vi "_OLS_5PtCalibration.vi"() -> ()   [LabVIEW 2024]
uses:
  Control Definitions/Def_PumpSpeed.ctl
  Control Definitions/DEF_CalConstants.ctl
  Control Definitions/Def PumpCtlRefs.ctl
  Control Definitions/Def CalTable.ctl
  Control Definitions/Def CalCoef.ctl
  Control Definitions/Def_LevelCalCoef.ctl
  Control Definitions/Registry Keys.ctl
  Control Definitions/Global 2.vi
  Control Definitions/Global 1.vi
  Control Definitions/DEF_5ptCalState.ctl
panel:
  out "Laser (raw) 2":dbl=-0.0 format="%#_4g"
  out "Numeric":i32
  out "Cal Coef":T1={"Level"={"M"=-0.9990777034816695, "B"=9.617362923679963, "Mc"=-1.0009231479344565, "Bc"=9.626241172397878, "LMe"=7.844}, "Dataq Ch"=[{"B"=-0.34241100677002123, "M"=175.4094780519764}, {"B"=-0.7865736704446391, "M"=174.89102005231038}]}
  in  "Default Cal Table":T3={"Level"={"LSf"=2.6, "LMf"=3.511, "LKf"=6.112, "LMe"=7.844, "LKe"=1.775, "LSe"=8.0}, "DataQ CH"=[{"RqLA"=0.592, "RmLA"=103.5, "RqHA"=5.171, "RmHA"=906.7}, {"RqLA"=0.582, "RmLA"=101.0, "RqHA"=5.17, "RmHA"=903.4}]}
  out "ItemPath":string
  in  "End Prog":bool
  out "PumpCtlRef out":T4
  out "Reg Cal Constants":T5={"Measure High"="3.125", "Laser High"="6.534", "Measure Low"="7.483", "Laser Low"="2.877", "Cal Name"="Rick A", "Cal Date"="8/22/2024 8:52:33 AM", "Empty Inches"=8.0, "Full Inches"=2.6, "Valid"=FALSE}
  in  "Pump Speed":T6=enum."STOP"
  in  "Num Chan":i32=2
  in  "VISA Refnum in":refnum<visa-resource-name>="COM3"
  in  "SimPV":bool
  out "Root Path":path=path "C:/AllenProjects/PWC-OLS"
  out "Time(ms)":dbl=1094.5499999995523
  out "Level":bool
  out "DataQ":bool
  in  "ChA":dbl(slide)=24.489795918367346 scale=0.0..1200.0
  in  "ChB":dbl(slide)=36.73469387755102 scale=0.0..1200.0
  in  "ChB +100":bool
  in  "ChA +100":bool
  in  "Check":bool
  out "Laser (raw)":dbl=-0.0 format="%#_4g"
  in  "DUT":i16=1
  in  "Pump JOG":bool=TRUE
  in  "Run Test":bool
  in  "Normal":cluster{u32, u32}[](array[cluster])=[{16711680, 1244948}]
  out "Level \nStatus":bool
  out "DataQ\nStatus":bool
  in  "Level SP":dbl(slide)=8.0 scale=8.5..2.0
  in  "Level PV":dbl(slide)=9.617362923679963 scale=8.5..2.0
  out "Level":dbl=9.617362923679963 format="%.3f"
  in  "Drain":bool
  in  "Fill":bool
  in  "Simulate":bool
  out "TEST NME":string="OLR001--"
  out "DataQ Input":T7(graph)={"ChA Ohms"=24.489795918367346, "ChB Ohms"=36.73469387755102, "Laser (raw)"=-0.0}
  out "Time Stamp":timestamp=timestamp(3809961154.032212 s since 1904-01-01)
  in  "stop":bool
  out "ChB Ohms":dbl=36.73469387755102 format="%.1f"
  out "ChA Ohms":dbl=24.489795918367346 format="%.1f"
  # "Calibration & Scaling Table\n               Tank         Key          Ref\n               Scale        Level        Measure\nEmpty\n\n\nFull"
  # "8.0      1.7752      7.844\n\n2.6      6.112        3.511"
  # "CHA"
  # "CHB"
  # "ATP       Resistance     Fill        Drain"
  # "ATP       Resistance     Fill        Drain"
  # "Simulated Instrument Inputs"
  # "PUMP"
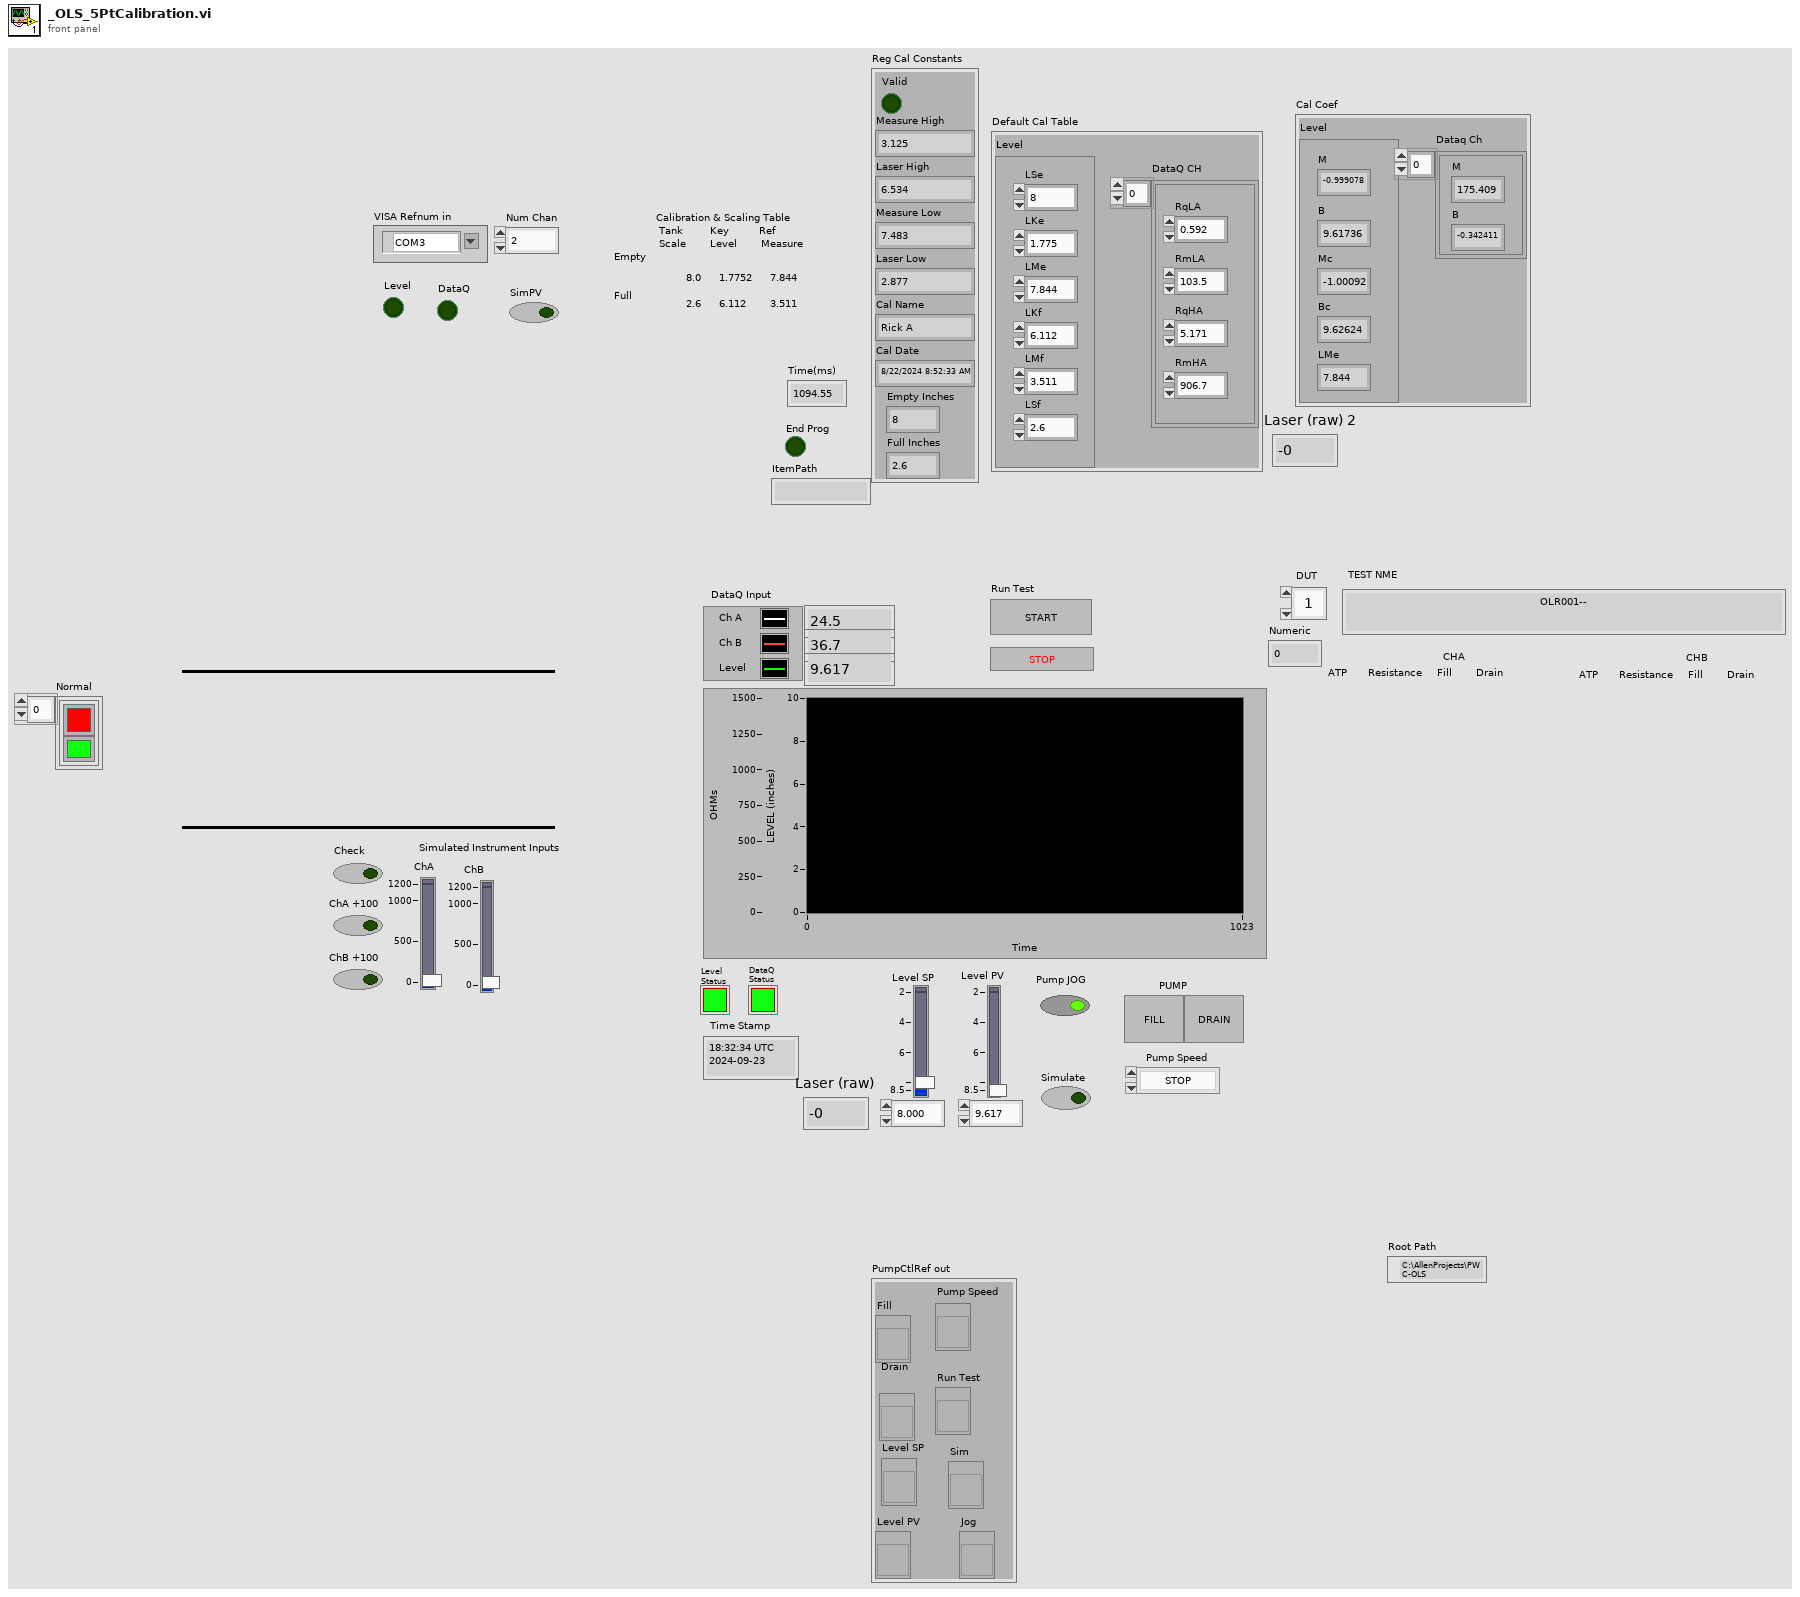
[diagram p1: front panel]
types:
  T1 = typedef "Def CalCoef.ctl" = cluster{"Level":T2, "Dataq Ch":cluster{"B":dbl, "M":dbl}[]}
  T2 = typedef "Def_LevelCalCoef.ctl" = cluster{"M":dbl, "B":dbl, "Mc":dbl, "Bc":dbl, "LMe":dbl}
  T3 = typedef "Def CalTable.ctl" = cluster{"Level":cluster{"LSf":dbl, "LMf":dbl, "LKf":dbl, "LMe":dbl, "LKe":dbl, "LSe":dbl}, "DataQ CH":cluster{"RqLA":dbl, "RmLA":dbl, "RqHA":dbl, "RmHA":dbl}[]}
  T4 = typedef "Def PumpCtlRefs.ctl" = cluster{"Fill ":refnum<vi>, "Drain":refnum<vi>, "Level PV":refnum<vi>, "Pump Speed":refnum<vi>, "Run Test":refnum<vi>, "Sim":refnum<vi>, "Jog":refnum<vi>, "Level SP":refnum<vi>}
  T5 = typedef "DEF_CalConstants.ctl" = cluster{"Measure High":string, "Laser High":string, "Measure Low":string, "Laser Low":string, "Cal Name":string, "Cal Date":string, "Empty Inches":dbl, "Full Inches":dbl, "Valid":bool}
  T6 = typedef "Def_PumpSpeed.ctl" = enum16{"FAST", "SLOW", "CREEP", "STOP"}
  T7 = cluster{"ChA Ohms":dbl, "ChB Ohms":dbl, "Laser (raw)":dbl}
  T8 = typedef "Registry Keys.ctl" = enum16{"Report Files Key", "Config Files Key"}
  T9 = cluster{"Level \nStatus":refnum<vi>, "DataQ\nStatus":refnum<vi>}
  T10 = typedef "Def FullCfg.ctl" = cluster{"Bench Config":T11, "Test Value Table ":dbl[][], "Table Col Titles":string[][], "cluster":T4, "Bench Status":T12}
  T11 = typedef "Def BenchCfg.ctl" = cluster{"Name":string, cluster{"Step Levels":dbl, "Tolerance":dbl, "Sample Rate":dbl, "Resistor":dbl, "M Level Cal":dbl, "[B Level Cal":dbl, "Max Fill Rate":dbl, "Empty Inches":dbl, "Full Inches":dbl}}
  T12 = typedef "Def Bench Status.ctl" = cluster{"Pump Status":refnum<vi>, "Instrumnet\n Status":refnum<vi>}
  T13 = typedef "DEF_5ptCalState.ctl" = enum16{"Start", "Load Tester", "Go Auto", "Level 1", "Reveiw ", "Save", "Exit"}
  T14 = cluster{"Resistor":dbl, "Fill":dbl, "Drain":dbl, "Status":i16}
  T15 = cluster{"Resistor":dbl, "Fill":dbl, "Drain":dbl, "Status":i16}[][]
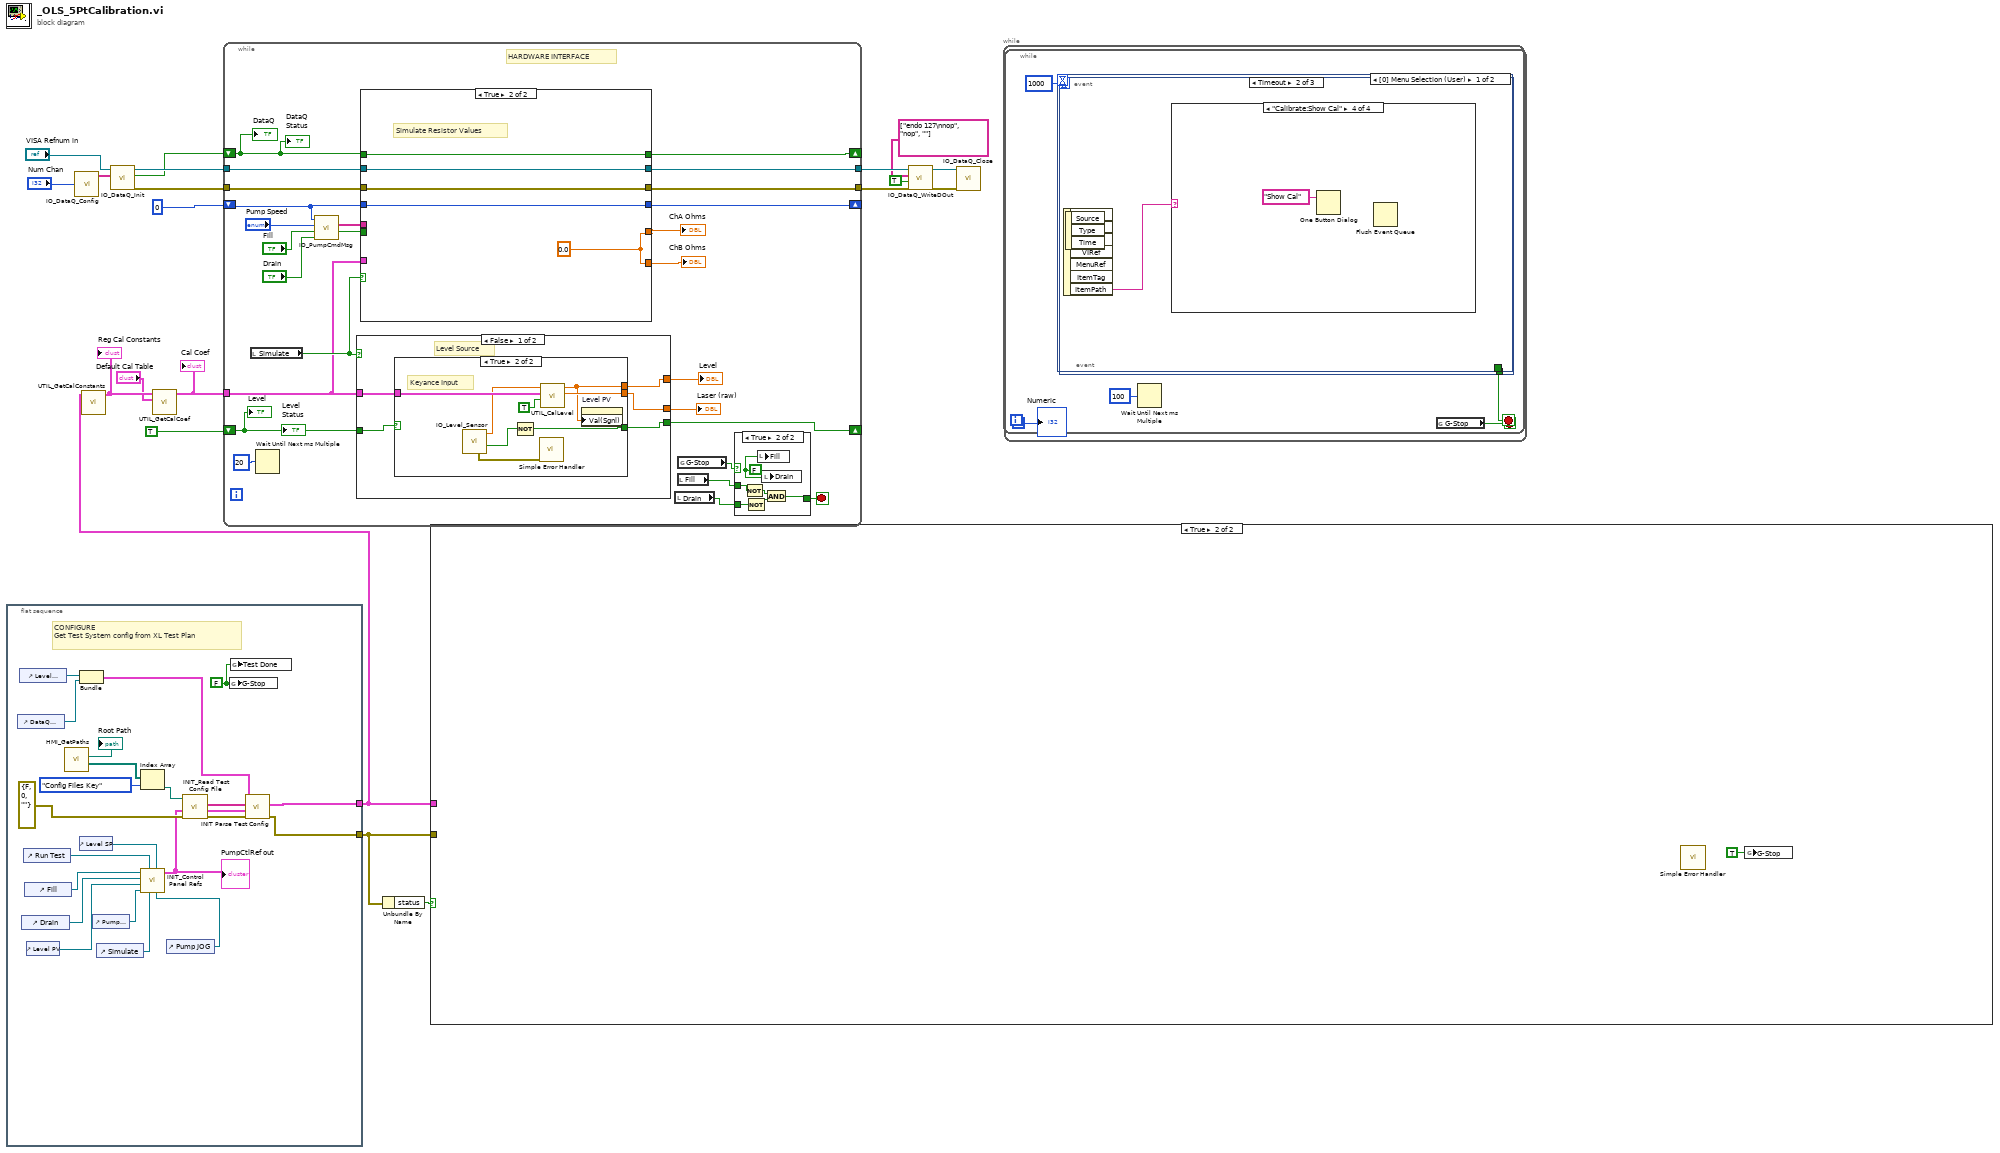
[diagram p0: block diagram]
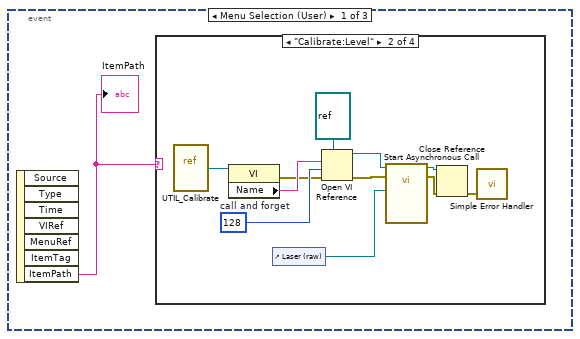
[diagram p2: hidden frame]
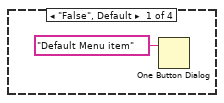
[diagram p3: hidden frame]
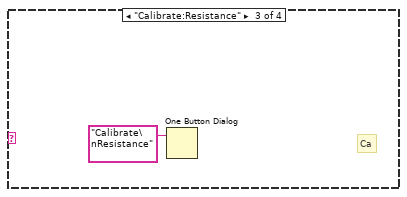
[diagram p4: hidden frame]
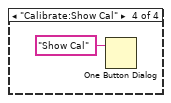
[diagram p5: hidden frame]
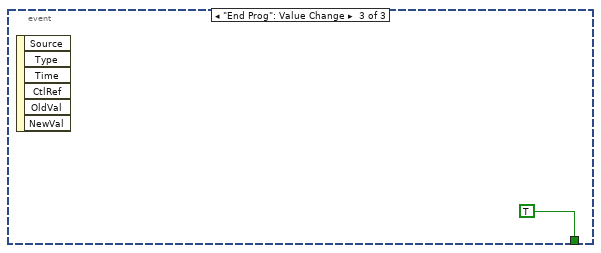
[diagram p6: hidden frame]
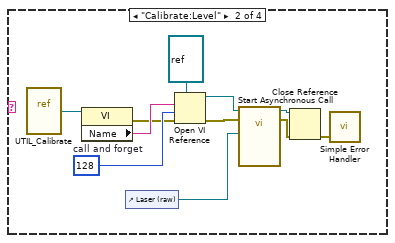
[diagram p8: hidden frame]
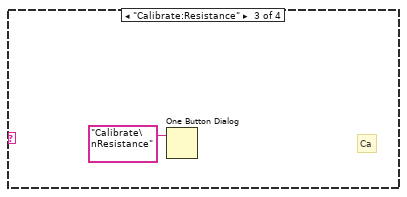
[diagram p9: hidden frame]
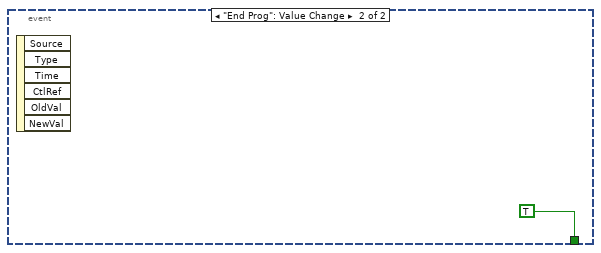
[diagram p10: hidden frame]
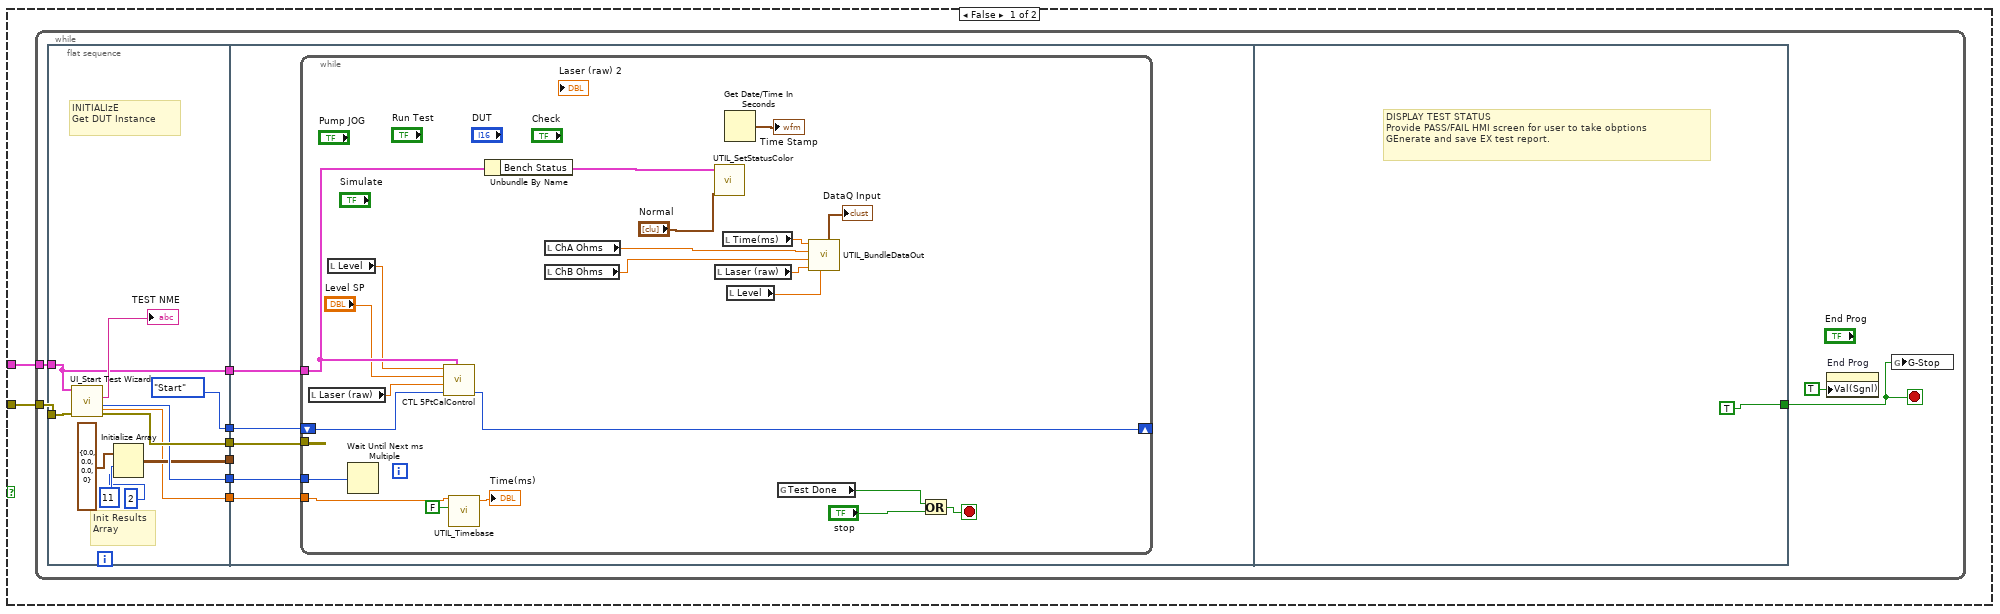
[diagram p11: hidden frame]
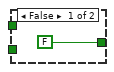
[diagram p12: hidden frame]
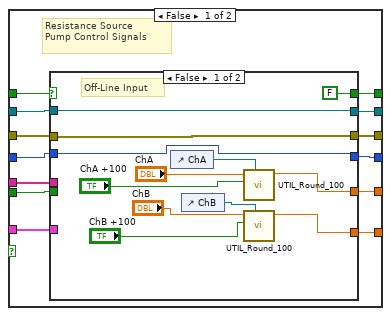
[diagram p13: hidden frame]
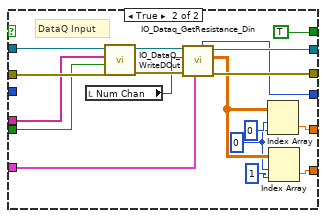
[diagram p14: hidden frame]
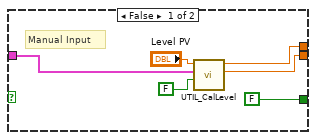
[diagram p15: hidden frame]
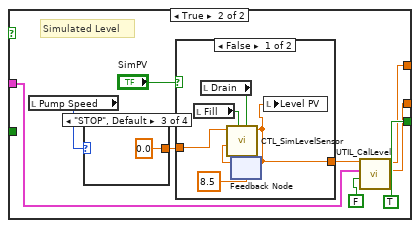
[diagram p16: hidden frame]
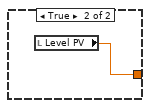
[diagram p17: hidden frame]
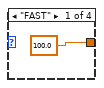
[diagram p18: hidden frame]
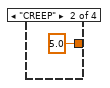
[diagram p19: hidden frame]
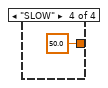
[diagram p20: hidden frame]
diagram:
  n1 = flat-sequence {
    tunnel: [w40] -> w14
    tunnel: [w32] -> w3
    frame #0 {
      w27 = FALSE ("G-Stop")
      # "CONFIGURE\nGet Test System config from XL Test Plan"
      n2 = control-ref of="DataQ\nStatus"() -> (w29:refnum<vi>)
      n3 = control-ref of="Level \nStatus"() -> (w39:refnum<vi>)
      n4 = control-ref of="Drain"() -> (w41:refnum<vi>)
      n5 = control-ref of="Run Test"() -> (w34:refnum<vi>)
      n6 = control-ref of="Fill"() -> (w35:refnum<vi>)
      n7 = control-ref of="Level PV"() -> (w37:refnum<vi>)
      n8 = call "HMI_GetPaths.vi"() -> ("Default Paths"=w22:path[], "Root Path"=→"Root Path":path)  [unwired: 10 in]
      n9 = Bundle("Level \nStatus"=w39, "DataQ\nStatus"=w29) -> (w38:T9)  [unwired: 1 in]
      n10 = control-ref of="Level SP"() -> (w28:refnum<vi>)
      n11 = control-ref of="Pump Speed"() -> (w24:refnum<vi>)
      n12 = control-ref of="Simulate"() -> (w31:refnum<vi>)
      n13 = Index Array(array=w22, index=Registry_Keys."Config Files Key" ("Reg Key")) -> (element=w21:path)
      n14 = control-ref of="Pump JOG"() -> (w30:refnum<vi>)
      n15 = call "INIT_Control Panel Refs.vi"("Jog"=w30, "Level SP"=w28, "Sim"=w31, "Run Test"=w34, "Pump Speed"=w24, "Level PV"=w37, "Drain"=w41, "Fill"=w35) -> ("PumpCtlRef out"=w25:T4)  [unwired: 3 in]
      "PumpCtlRef out" <- w25
      n16 = call "INIT_Read Test Config File.vi"("error in (no error)"=errorcluster {"status"=FALSE, "code"=0, "source"=""}, "Path"=w21) -> ("error out 2"=w33:errorcluster, "Config\nFile Data"=w36:string[][])  [unwired: 8 in]
      n17 = global write "Global 1.vi" "G-Stop"(w27) -> ()
      n18 = global write "Global 2.vi" "Test Done"(w27) -> ()
      n19 = call "INIT Parse Test Config.vi"("error in (no error)"=w33, "Pump CtlRef In"=w25, "All XL Input"=w36, "Bench Status"=w38) -> ("error out"=w40:errorcluster, "Full Config"=w32:T10)  [unwired: 5 in, 1 out]
    }
  }
  n20 = call "IO_DataQ_Config.vi"("Num Chan"="Num Chan") -> ("Init Message"=w20:string[])  [unwired: 10 in]
  n21 = call "UTIL_GetCalConstants.vi"("Full Config"=w3) -> ("Cal Constants"=w4:T5)  [unwired: 9 in, 1 out]
  "Reg Cal Constants" <- w4
  n22 = call "IO_DataQ_Init.vi"("Command\nList"=w20, "VISA Refnum in"="VISA Refnum in") -> ("error out"=w18:errorcluster, "Connected?"=w17:bool, "VISA resource name out"=w19:refnum<visa-resource-name>)  [unwired: 7 in]
  n23 = call "UTIL_GetCalCoef.vi"("Cal Table"="Default Cal Table", "Cal Constants"=w4) -> ("Cal Coef"=w1:T1)  [unwired: 9 in]
  "Cal Coef" <- w1
  n24 = while {
    shift-right: [w65] -> _
    shift-left: TRUE ("Pump \nStatus") -> [w47]
    tunnel: w19 -> [w64]
    tunnel: w18 -> [w63]
    tunnel: [w61] -> w13
    tunnel: [w62] -> w11
    shift-right: [w60] -> _
    shift-left: w17 -> [w59]
    tunnel: w1 -> [w43]
    shift-right: [w50] -> _
    shift-left: 0 -> [w46]
    stop <- w55 stop-if-true
    # "HARDWARE INTERFACE"
    n25 = local read "Simulate"() -> (w57:bool)
    n26 = Wait Until Next ms Multiple(millisecond multiple=u32 20) -> ()  [unwired: 1 out]
    n27 = call "IO_PumpCmdMsg.vi"("Drain Signal"="Drain", "FIll Signal"="Fill", "Pump Speed"="Pump Speed", "Cmd IN"=w46) -> ("Msg Active"=w44:bool, "Message"=w58:string[])  [unwired: 4 in, 2 out]
    n28 = case shown="False" w57 {
      tunnel: [w128 w148] -> w45
      tunnel: [w127 w150] -> w66
      tunnel: [w124 TRUE] -> w65
      tunnel: w47 -> [w126 _]
      tunnel: w43 -> [w125 w143]
      frame False {
        # "Level Source"
        n29 = case shown="True" w126 {
          tunnel: [w132 w135] -> w128
          tunnel: [w131 w140] -> w127
          tunnel: [FALSE ("status") w139] -> w124
          tunnel: w125 -> [w133 w141]
          frame False {
            # "Manual Input"
            n30 = call "UTIL_CalLevel.vi"("Key is In?"=FALSE, "Cal Coef"=w133, "Input"="Level PV") -> ("PVc"=w131:dbl, "PVs"=w132:dbl)  [unwired: 7 in]
          }
          frame True {
            # "Keyance Input"
            n31 = call "IO_Level_Sensor.vi"() -> ("status"=w137:bool, "PV (raw)"=w138:dbl, "error OUT"=w136:errorcluster)  [unwired: 9 in]
            n32 = Not(x=w137) -> (.not. x?=w139:bool)
            n33 = call <vilib>:"Simple Error Handler.vi"("error in (no error)"=w136) -> ()  [unwired: 4 in, 5 out]
            n34 = call "UTIL_CalLevel.vi"("Key is In?"=TRUE, "Cal Coef"=w141, "Input"=w138) -> ("PVc"=w140:dbl, "PVs"=w135:dbl)  [unwired: 7 in]
            n35 = property on="Level PV" class="Slide (strict)"("Val(Sgnl)"=w135) -> ()  [unwired: 2 in, 2 out]
          }
        }
      }
      frame True {
        # "Simulated Level"
        n36 = local read "Pump Speed"() -> (w146:T6)
        n37 = case shown="\"STOP\", Default" w146 {
          tunnel: [100.0 ("Ctl Sig") 5.0 ("Ctl Sig") 0.0 ("Ctl Sig") 50.0 ("Ctl Sig")] -> w147
          frame "FAST" {
          }
          frame "CREEP" {
          }
          frame "STOP", Default {
          }
          frame "SLOW" {
          }
        }
        n38 = case shown="False" "SimPV" {
          tunnel: w147 -> [w156 _]
          tunnel: [w152 w158] -> w145
          frame False {
            n39 = local read "Fill"() -> (w157:bool)
            n40 = local read "Drain"() -> (w153:bool)
            n41 = feedback #1(8.5 ("PV Level Inch")) -> (w154:dbl)
            n42 = call "CTL_SimLevelSensor.vi"("Drain IN"=w153, "Fill IN"=w157, "Level PV in"=w154, "Pump Speed"=w156) -> ("PV Level Inch"=w152:dbl)  [unwired: 7 in]
            n43 = feedback-in #1(w152) -> ()
            n44 = local write "Level PV"(w152) -> ()
          }
          frame True {
            n45 = local read "Level PV"() -> (w158:dbl)
          }
        }
        n46 = call "UTIL_CalLevel.vi"("Key is In?"=FALSE, "Cal Coef"=w143, "Input"=w145) -> ("PVc"=w150:dbl, "PVs"=w148:dbl)  [unwired: 7 in]
      }
    }
    "Level" <- w45
    "Laser (raw)" <- w66
    n47 = case shown="True" w57 {
      tunnel: [w88 w119] -> w67
      tunnel: [w87 w119] -> w48
      tunnel: w64 -> [w80 w122]
      tunnel: w63 -> [w82 w121]
      tunnel: [w86 w121] -> w62
      tunnel: [w85 w122] -> w61
      tunnel: [w84 w123] -> w60
      tunnel: w59 -> [w83 w123]
      tunnel: w58 -> [w81 _]
      tunnel: w44 -> [w79 _]
      tunnel: [w78 w120] -> w50
      tunnel: w46 -> [w77 w120]
      tunnel: w43 -> [w76 _]
      frame False {
        # "Resistance Source\nPump Control Signals"
        n48 = case shown="False" w83 {
          tunnel: [w93 w115] -> w88
          tunnel: [w94 w104] -> w87
          tunnel: [w95 w118] -> w85
          tunnel: [w96 w117] -> w86
          tunnel: [FALSE TRUE] -> w84
          tunnel: w82 -> [w96 w113]
          tunnel: w81 -> [_ w109]
          tunnel: w80 -> [w95 w112]
          tunnel: w79 -> [_ w108]
          tunnel: [w89 w105] -> w78
          tunnel: w77 -> [w89 _]
          tunnel: w76 -> [_ w101]
          frame False {
            # "Off-Line Input"
            n49 = control-ref of="ChA"() -> (w92:refnum<vi>)
            n50 = control-ref of="ChB"() -> (w90:refnum<vi>)
            n51 = call "UTIL_Round_100.vi"("Num Refnum"=w92, "100"="ChA +100", "IN"="ChA") -> ("OUT"=w94:dbl)  [unwired: 8 in]
            n52 = call "UTIL_Round_100.vi"("Num Refnum"=w90, "100"="ChB +100", "IN"="ChB") -> ("OUT"=w93:dbl)  [unwired: 8 in]
          }
          frame True {
            w103 = 0 ("disabled index (col)")
            # "DataQ Input"
            n53 = local read "Num Chan"() -> (w106:i32)
            n54 = call "IO_DataQ_WriteDOut.vi"("error in (no error)"=w113, "Msg Active"=w108, "Message"=w109, "VISA Refnum in"=w112) -> ("error out"=w111:errorcluster, "VISA Refnum out"=w110:refnum<visa-resource-name>)  [unwired: 6 in]
            n55 = call "IO_Dataq_GetResistance_Din.vi"("Cal Coef"=w101, "error in (no error)"=w111, "Num Chan"=w106, "VISA Refnum in"=w110) -> ("error out"=w117:errorcluster, "Analog"=w107:dbl[][], "VISA Refnum out"=w118:refnum<visa-resource-name>, "Cmd"=w105:u32)  [unwired: 2 in, 2 out]
            n56 = Index Array(array=w107, index (row)=0 ("index"), index (col)=w103) -> (element=w104:dbl)
            n57 = Index Array(array=w107, index (row)=w103, index (col)=1 ("index")) -> (element=w115:dbl)
          }
        }
      }
      frame True {
        w119 = 0.0 ("OUT")
        # "Simulate Resistor Values"
      }
    }
    "ChA Ohms" <- w48
    "ChB Ohms" <- w67
    n58 = local read "Drain"() -> (w53:bool)
    n59 = local read "Fill"() -> (w54:bool)
    n60 = global read "Global 1.vi" "G-Stop"() -> (w56:bool)
    n61 = case shown="True" w56 {
      tunnel: [FALSE w71] -> w55
      tunnel: w54 -> [_ w73]
      tunnel: w53 -> [_ w70]
      frame False {
      }
      frame True {
        w75 = FALSE
        n62 = Not(x=w73) -> (.not. x?=w74:bool)
        n63 = Not(x=w70) -> (.not. x?=w72:bool)
        n64 = local write "Fill"(w75) -> ()
        n65 = local write "Drain"(w75) -> ()
        n66 = And(x=w74, y=w72) -> (x .and. y?=w71:bool)
      }
    }
    "DataQ\nStatus" <- w59
    "Level \nStatus" <- w47
    "DataQ" <- w59
    "Level" <- w47
  }
  n67 = Unbundle By Name(w14) -> ("status"=w16:bool)
  n68 = case shown="True" w16 {
    tunnel: w14 -> [w164 _]
    tunnel: w3 -> [w163 _]
    frame False {
      n69 = while {
        tunnel: w164 -> [w172]
        tunnel: w163 -> [w170]
        stop <- w166 stop-if-true
        n70 = flat-sequence {
          tunnel: [w183] -> w174
          tunnel: [w184] -> w173
          tunnel: w172 -> [w185]
          tunnel: [w176] -> w171
          tunnel: w170 -> [w176]
          tunnel: [DEF_5ptCalState."Start" ("Cal State In")] -> w169
          tunnel: [w178] -> w168
          tunnel: [w177] -> w167
          tunnel: w174 -> [w189]
          tunnel: w173 -> [w190]
          tunnel: w171 -> [w186]
          tunnel: w169 -> [w187]
          tunnel: w168 -> [_]
          tunnel: w167 -> [w188]
          tunnel: [TRUE] -> w166
          frame #0 {
            # "Init Results\nArray"
            # "INITIALIzE\nGet DUT Instance"
            n71 = call "UI_Start Test Wizard.vi"("error in (no error)"=w185, "Full Config"=w176) -> ("error out"=w184:errorcluster, "Time Base mS"=w183:i32, "Title"=→"TEST NME":string, "Sample Rate"=w177:dbl)  [unwired: 4 in]
            n72 = Initialize Array(T14 {"Resistor"=0.0, "Fill"=0.0, "Drain"=0.0, "Status"=0} ("Cluster 2"), 11 ("dimension size"), 2 ("dimension size")) -> (w178:T15)
          }
          frame #1 {
            n73 = while {
              tunnel: w189 -> [w211]
              tunnel: w190 -> [_]
              tunnel: w188 -> [w201]
              shift-right: [w193] -> _
              shift-left: w187 -> [w194]
              tunnel: w186 -> [w197]
              stop <- w208 stop-if-true
              n74 = local read "Laser (raw)"() -> (w191:dbl)
              n75 = local read "Level"() -> (w196:dbl)
              n76 = Wait Until Next ms Multiple(millisecond multiple=w211) -> ()  [unwired: 1 out]
              n77 = call "CTL 5PtCalControl.vi"("Full Cfg 2"=w197, "Cal State In"=w194, "Laser Raw"=w191, "Level SP"="Level SP", "Level PV"=w196) -> ("Cal State Out"=w193:T13)  [unwired: 6 in]
              n78 = call "UTIL_Timebase.vi"("Reset"=FALSE, "Sample Rate"=w201) -> ("Time(ms)"=→"Time(ms)":dbl)  [unwired: 9 in]
              n79 = Unbundle By Name(w197) -> ("Bench Status"=w209:T12)
              n80 = local read "ChA Ohms"() -> (w203:dbl)
              n81 = local read "ChB Ohms"() -> (w202:dbl)
              n82 = call "UTIL_SetStatusColor.vi"("Colors [4] in"="Normal", "Bench Status"=w209) -> ()  [unwired: 10 in]
              n83 = local read "Laser (raw)"() -> (w204:dbl)
              n84 = local read "Time(ms)"() -> (w205:dbl)
              n85 = Get Date/Time In Seconds() -> (seconds since 1Jan1904=→"Time Stamp":timestamp)
              n86 = local read "Level"() -> (w198:dbl)
              n87 = global read "Global 2.vi" "Test Done"() -> (w206:bool)
              n88 = call "UTIL_BundleDataOut.vi"("Level PV"=w198, "Laser (raw)"=w204, "ChB Ohms"=w202, "ChA Ohms"=w203, "Time (ms)"=w205) -> ("Chart Data"=→"DataQ Input":T7)  [unwired: 3 in, 3 out]
              n89 = Or(x=w206, y="stop") -> (x .or. y?=w208:bool)
            }
          }
          frame #2 {
            # "DISPLAY TEST STATUS\nProvide PASS/FAIL HMI screen for user to take obptions\nGEnerate and save EX test report."
          }
        }
        n90 = property on="End Prog" class="Bool (strict)"("Val(Sgnl)"=TRUE ("End Prog")) -> ()  [unwired: 2 in, 2 out]
        n91 = global write "Global 1.vi" "G-Stop"(w166) -> ()
      }
    }
    frame True {
      n92 = call <vilib>:"Simple Error Handler.vi"() -> ()  [unwired: 5 in, 5 out]
      n93 = global write "Global 1.vi" "G-Stop"(TRUE ("G-Stop")) -> ()
    }
  }
  n94 = call "IO_DataQ_WriteDOut.vi"("error in (no error)"=w11, "Msg Active"=TRUE, "Message"=string[] ["endo 127\nnop", "nop", ""], "VISA Refnum in"=w13) -> ("error out"=w10:errorcluster, "VISA Refnum out"=w12:refnum<visa-resource-name>)  [unwired: 6 in]
  n95 = call "IO_DataQ_Close.vi"("error in"=w10, "VISA resource name"=w12) -> ()  [unwired: 10 in]
  n96 = while {
    stop <- w215 stop-if-true
    n97 = event shown="[0] Menu Selection (User)" {
      selector: _ -> [_ _]
      dyn-events: _ -> [_ _]
      timeout: _ -> [_ _]
      tunnel: [_ TRUE] -> w215
      event Menu Selection (User) {
        n98 = event-data() -> ("ItemPath"=w216:string)  [unwired: 1 in, 6 out]
        n99 = case shown="\"Calibrate:Show Cal\"" w216 {
          frame "False", Default {
          }
          frame "Calibrate:Level" {
            w227 = 128  # call and forget
            n100 = vi-ref "UTIL_Calibrate.vi"() -> (w220:refnum<vi>)
            n101 = property class="VI"(reference=w220) -> (error out=w218:errorcluster, "Name"=w219:string)  [unwired: 1 in, 1 out]
            n102 = control-ref of="Laser (raw)"() -> (w217:refnum<vi>)
            n103 = Open VI Reference(type specifier VI Refnum (for type only)=refnum<vi> refnum, vi path=w219, options=w227, error in (no error)=w218) -> (vi reference=w225:refnum<vi>, error out=w224:errorcluster)  [unwired: 2 in]
            n104 = call-by-ref "Start Asynchronous Call"(reference=w225, error in=w224, "Digital in"=w217) -> (reference out=w222:refnum<vi>, error out=w223:errorcluster)  [unwired: 10 in, 1 out]
            n105 = Close Reference(reference=w222, error in (no error)=w223) -> (error out=w221:errorcluster)
            n106 = call <vilib>:"Simple Error Handler.vi"("error in (no error)"=w221) -> ()  [unwired: 4 in, 5 out]
          }
          frame "Calibrate:Resistance" {
            # "Ca"
            n107 = One Button Dialog(message="Calibrate\nResistance") -> ()  [unwired: 1 in, 1 out]
          }
          frame "Calibrate:Show Cal" {
            n108 = One Button Dialog(message="Show Cal") -> ()  [unwired: 1 in, 1 out]
          }
        }
      }
      event "End Prog": Value Change {
        n109 = event-data() -> ()  [unwired: 1 in, 6 out]
      }
    }
  }
  n110 = while {
    i -> [w232]
    stop <- w231 stop-if-true
    n111 = event shown="[1] Timeout" {
      selector: _ -> [_ _ _]
      dyn-events: _ -> [_ _ _]
      timeout: 1000 -> [_ _ _]
      tunnel: [_ _ TRUE] -> _
      event Menu Selection (User) {
        n112 = event-data() -> ("ItemPath"=w235:string)  [unwired: 1 in, 6 out]
        "ItemPath" <- w235
        n113 = case shown="\"Calibrate:Level\"" w235 {
          frame "False", Default {
            n114 = One Button Dialog(message="Default Menu item") -> ()  [unwired: 1 in, 1 out]
          }
          frame "Calibrate:Level" {
            w247 = 128  # call and forget
            n115 = vi-ref "UTIL_Calibrate.vi"() -> (w240:refnum<vi>)
            n116 = property class="VI"(reference=w240) -> (error out=w238:errorcluster, "Name"=w239:string)  [unwired: 1 in, 1 out]
            n117 = control-ref of="Laser (raw)"() -> (w237:refnum<vi>)
            n118 = Open VI Reference(type specifier VI Refnum (for type only)=refnum<vi> refnum, vi path=w239, options=w247, error in (no error)=w238) -> (vi reference=w245:refnum<vi>, error out=w244:errorcluster)  [unwired: 2 in]
            n119 = call-by-ref "Start Asynchronous Call"(reference=w245, error in=w244, "Digital in"=w237) -> (reference out=w242:refnum<vi>, error out=w243:errorcluster)  [unwired: 10 in, 1 out]
            n120 = Close Reference(reference=w242, error in (no error)=w243) -> (error out=w241:errorcluster)
            n121 = call <vilib>:"Simple Error Handler.vi"("error in (no error)"=w241) -> ()  [unwired: 4 in, 5 out]
          }
          frame "Calibrate:Resistance" {
            # "Ca"
            n122 = One Button Dialog(message="Calibrate\nResistance") -> ()  [unwired: 1 in, 1 out]
          }
          frame "Calibrate:Show Cal" {
            n123 = One Button Dialog(message="Show Cal") -> ()  [unwired: 1 in, 1 out]
          }
        }
      }
      event Timeout {
        n124 = event-data() -> ()  [unwired: 1 in, 3 out]
        n125 = Flush Event Queue() -> ()  [unwired: 6 in, 3 out]
      }
      event "End Prog": Value Change {
        n126 = event-data() -> ()  [unwired: 1 in, 6 out]
      }
    }
    n127 = Wait Until Next ms Multiple(millisecond multiple=u32 100) -> ()  [unwired: 1 out]
    n128 = global read "Global 1.vi" "G-Stop"() -> (w231:bool)
    "Numeric" <- w232
  }
